vi "M_Series_Change_Detection_Event.vi"() -> ()   [LabVIEW 2015]
doc: "-----------------------------\nHardware Requirements\n-----------------------------\nAny M Series board and an external digital connection to monitor.\n\n-----------------------------\nVI Description\n-----------------------------\n\nThis example shows how to use an M Series multi-function DAQ board and DAQmx Events to execute code upon a digital change detection event.\n\nIn order to function, this example requires both LabVIEW 8.0 and NI-DAQmx 8.0 or later. Change Detection was not supported for M Series prior to NI-DAQmx 8.0\n\nPort 0 of the M Series board must be used for the Change Detection Lines.\n\n-----------------------------\nBlock Diagram Steps\n-----------------------------\n\n1. Create a Digital Input Channel using the indicated Digital Input Lines\n2. Configure the task for Change Detection Timing with the indicated Change Detection Lines\n3. Register the \"Signal\" DAQmx Event for the Change Detection Event Signal Type.\n4. Start the task.\n5. Display current Changes Detected count\n6. Increment the Changes Detected count in the case of a Change Detection Event occurrence.\n7. Clear the task and handle any errors."
uses:
  <vilib>/DAQmx/create/channels.llb/DAQmx Create Channel (DI-Digital Input).vi
  <vilib>/DAQmx/configure/timing.llb/DAQmx Timing (Change Detection).vi
panel:
  in  "stop":bool
  out "Changes Detected":i32=2
  in  "Change Detection Lines":tag="PXI1Slot4/port0/line0"
  in  "Digital Input Lines":tag="PXI1Slot4/port0/line0"
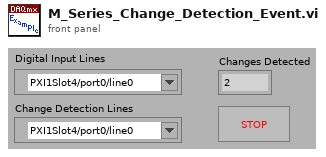
[diagram p1: front panel]
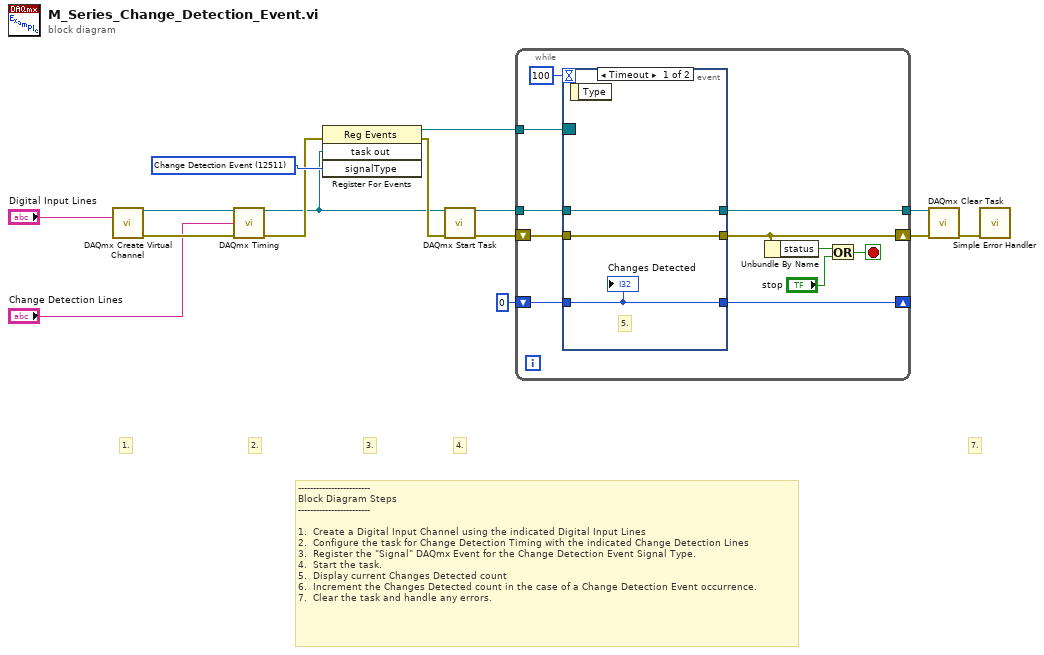
[diagram p0: block diagram]
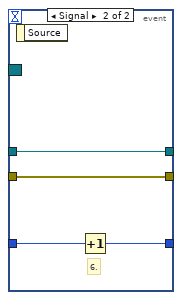
[diagram p2: hidden frame]
diagram:
  w11 = 12511 items=["Sample Complete Event"=12530, "Counter Output Event"=12494, "Change Detection Event"=12511, "Sample Clock"=12487] ("signalType")
  # "------------------------\nBlock Diagram Steps\n------------------------\n\n1.  Create a Digital Input Channel using the indicated Digital Input Lines\n2.  Configure the task for Change Detection Timing with the indicated Change Detection Lines\n3.  Register the \"Signal\" DAQmx Event for the Change Detection Event Signal Type.\n4.  Start the task.\n5.  Display current Changes Detected count\n6.  Increment the Changes Detected count in the case of a Change Detection Event occurrence.\n7.  Clear the task and handle any errors."
  # "7."
  # "4."
  # "3."
  # "2."
  # "1."
  n1 = call-poly <vilib>:"DAQmx Create Virtual Channel.vi"("lines"="Digital Input Lines") -> ("task out"=w13:refnum<k21>, "error out"=w14:errorcluster)  [unwired: 13 in]
  n2 = call-poly <vilib>:"DAQmx Timing.vi"("task/channels in"=w13, "rising edge physical channels"="Change Detection Lines", "error in"=w14) -> ("task out"=w8:refnum<k21>, "error out"=w10:errorcluster)  [unwired: 11 in]
  n3 = register-events(error in=w10, w8, w11) -> (reference out=w7:refnum<event-registration>, error out=w9:errorcluster)  [unwired: 1 in]
  n4 = call <vilib>:"DAQmx Start Task.vi"("task/channels in"=w8, "error in"=w9) -> ("task out"=w6:refnum<k21>, "error out"=w5:errorcluster)  [unwired: 12 in]
  n5 = while {
    tunnel: w7 -> [w26]
    tunnel: w6 -> [w24]
    tunnel: [w22] -> w3
    shift-right: [w20] -> _
    shift-left: 0 -> [w21]
    shift-right: [w19] -> w2
    shift-left: w5 -> [w23]
    stop <- w16 stop-if-true
    n6 = event shown="[0] Timeout" {
      selector: w26 -> [_ _]
      dyn-events: _ -> [_ _]
      timeout: 100 -> [_ _]
      tunnel: w24 -> [w29 w33]
      tunnel: w23 -> [w28 w32]
      tunnel: [w29 w33] -> w22
      tunnel: [w28 w32] -> w19
      tunnel: w21 -> [w27 w31]
      tunnel: [w27 w30] -> w20
      event Timeout {
        # "5."
        n7 = event-data() -> ()  [unwired: 1 in, 1 out]
        "Changes Detected" <- w27
      }
      event Signal {
        # "6."
        n8 = event-data() -> ()  [unwired: 1 in, 1 out]
        n9 = Increment(x=w31) -> (x+1=w30:i32)
      }
    }
    n10 = Unbundle By Name(w19) -> ("status"=w18:bool)
    n11 = Or(x=w18, y="stop") -> (x .or. y?=w16:bool)
  }
  n12 = call <vilib>:"DAQmx Clear Task.vi"("task in"=w3, "error in"=w2) -> ("error out"=w1:errorcluster)  [unwired: 13 in]
  n13 = call <vilib>:"Simple Error Handler.vi"("error in (no error)"=w1) -> ()  [unwired: 4 in, 5 out]
